vi "arithmetic operations.vi"() -> ()   [LabVIEW 2017]
panel:
  out "floor(x/y) 2":dbl
  out "floor(x/y)":dbl
  out "DIVIDE":dbl(slide) scale=0.0..10.0
  out "MULTIPLY":dbl(slide) scale=0.0..2000.0
  out "SUBTRACT":dbl(slide) scale=0.0..100.0
  out "ADD":dbl(slide) scale=0.0..200.0
  in  "INPUT2":dbl(knob) scale=0.0..100.0
  in  "INTPUT1":dbl(knob) scale=0.0..100.0
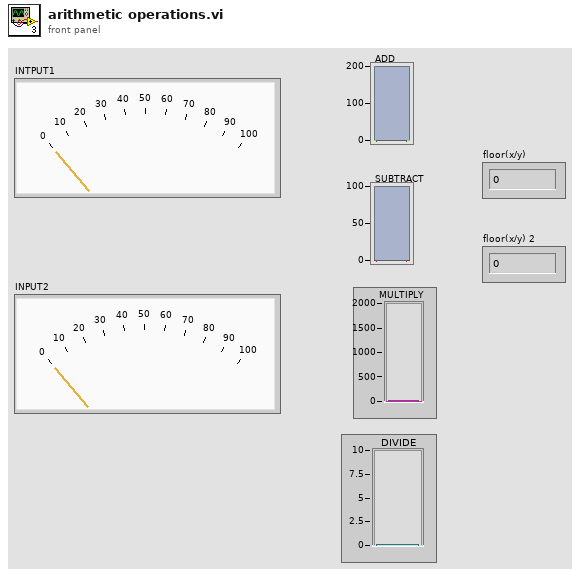
[diagram p1: front panel]
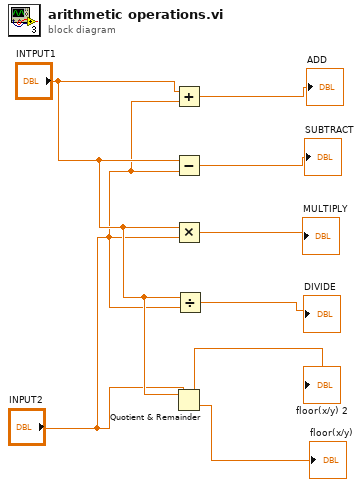
[diagram p0: block diagram]
diagram:
  n1 = Add(x="INTPUT1", y="INPUT2") -> (x+y=→"ADD":dbl)
  n2 = Subtract(x="INTPUT1", y="INPUT2") -> (x-y=→"SUBTRACT":dbl)
  n3 = Multiply(x="INTPUT1", y="INPUT2") -> (x*y=→"MULTIPLY":dbl)
  n4 = Quotient & Remainder(x="INTPUT1", y="INPUT2") -> (x-y*floor(x/y)=→"floor(x/y) 2":dbl, floor(x/y)=→"floor(x/y)":dbl)
  n5 = Divide(x="INTPUT1", y="INPUT2") -> (x/y=→"DIVIDE":dbl)
